vi "2013_01_03 Quality Motor.vi"(8 "Capture":bool, 9 "data":waveform(dbl)[](array[waveform]), 10 "File Path":path, 11 "Motor Typedef":T1={"Write"=FALSE, "Fail"=FALSE, "RPM"=0, "Motor"=enum."Maxon EC6 6V", "ESC"=enum."Phoenix", "Supply (V)"=0.0, "Test ID and Serial #"="", "Comments"="", "Elapsed Time"=0.0, "Counter"=0.0, "Torque (mNm)"=0.0, "Electrical Power (W)"=0.0, "Motor Efficiency"=0.0, "Mechanical Power (W)"=0.0, "Supply Power (W)"=0.0, "ESC Efficiency"=0.0, "No Load Speed"=0, "Stall Torque"=0.0, "Speed/Torque Gradient"=0, "Calcul"=FALSE, "Clear"=FALSE, "No Load Torque"=0.0} {"No Load Torque" format="%.3f"; "Stall Torque" format="%.3f"; "ESC Efficiency" format="%#_3g%%"; "Supply Power (W)" format="%.3f"; "Mechanical Power (W)" format="%.3f"; "Motor Efficiency" format="%#_3g%%"; "Electrical Power (W)" format="%.3f"; "Torque (mNm)" format="%.3f"; "Elapsed Time" format="%<%H:%M:%S>t"; "Supply (V)" format="%.2f"; "RPM" scale=0.0..60000.0}) -> (0 "Final Out":dynamicdata(graph), 3 "Motor Typedef Out":T1={"Write"=FALSE, "Fail"=FALSE, "RPM"=0, "Motor"=enum."Maxon EC6 6V", "ESC"=enum."Phoenix", "Supply (V)"=0.0, "Test ID and Serial #"="", "Comments"="", "Elapsed Time"=0.0, "Counter"=0.0, "Torque (mNm)"=0.0, "Electrical Power (W)"=0.0, "Motor Efficiency"=0.0, "Mechanical Power (W)"=0.0, "Supply Power (W)"=0.0, "ESC Efficiency"=0.0, "No Load Speed"=0, "Stall Torque"=0.0, "Speed/Torque Gradient"=0, "Calcul"=FALSE, "Clear"=FALSE, "No Load Torque"=0.0} {"No Load Torque" format="%.3f"; "Stall Torque" format="%.3f"; "ESC Efficiency" format="%#_3g%%"; "Supply Power (W)" format="%.3f"; "Mechanical Power (W)" format="%.3f"; "Motor Efficiency" format="%#_3g%%"; "Electrical Power (W)" format="%.3f"; "Torque (mNm)" format="%.3f"; "Elapsed Time" format="%<%H:%M:%S>t"; "Supply (V)" format="%.2f"; "RPM" scale=0.0..60000.0})   [LabVIEW 2013]
uses:
  Quality Type Def.ctl
  <vilib>/express/express shared/transition.llb/Dynamic To Waveform Array.vi
  <vilib>/express/express signal manip/GetorSetDDTAttributes/Set DDT Attributes/SetT0.vi
  <vilib>/express/express shared/transition.llb/Waveform Array To Dynamic.vi
  <vilib>/express/express signal manip/GetorSetDDTAttributes/Set DDT Attributes/Set DDT Properties.xnode
panel:
  in  "error in (no error)":errorcluster
  out "error out":errorcluster
  out "Saving Data":bool
  # "Fail"
  # "Fail"
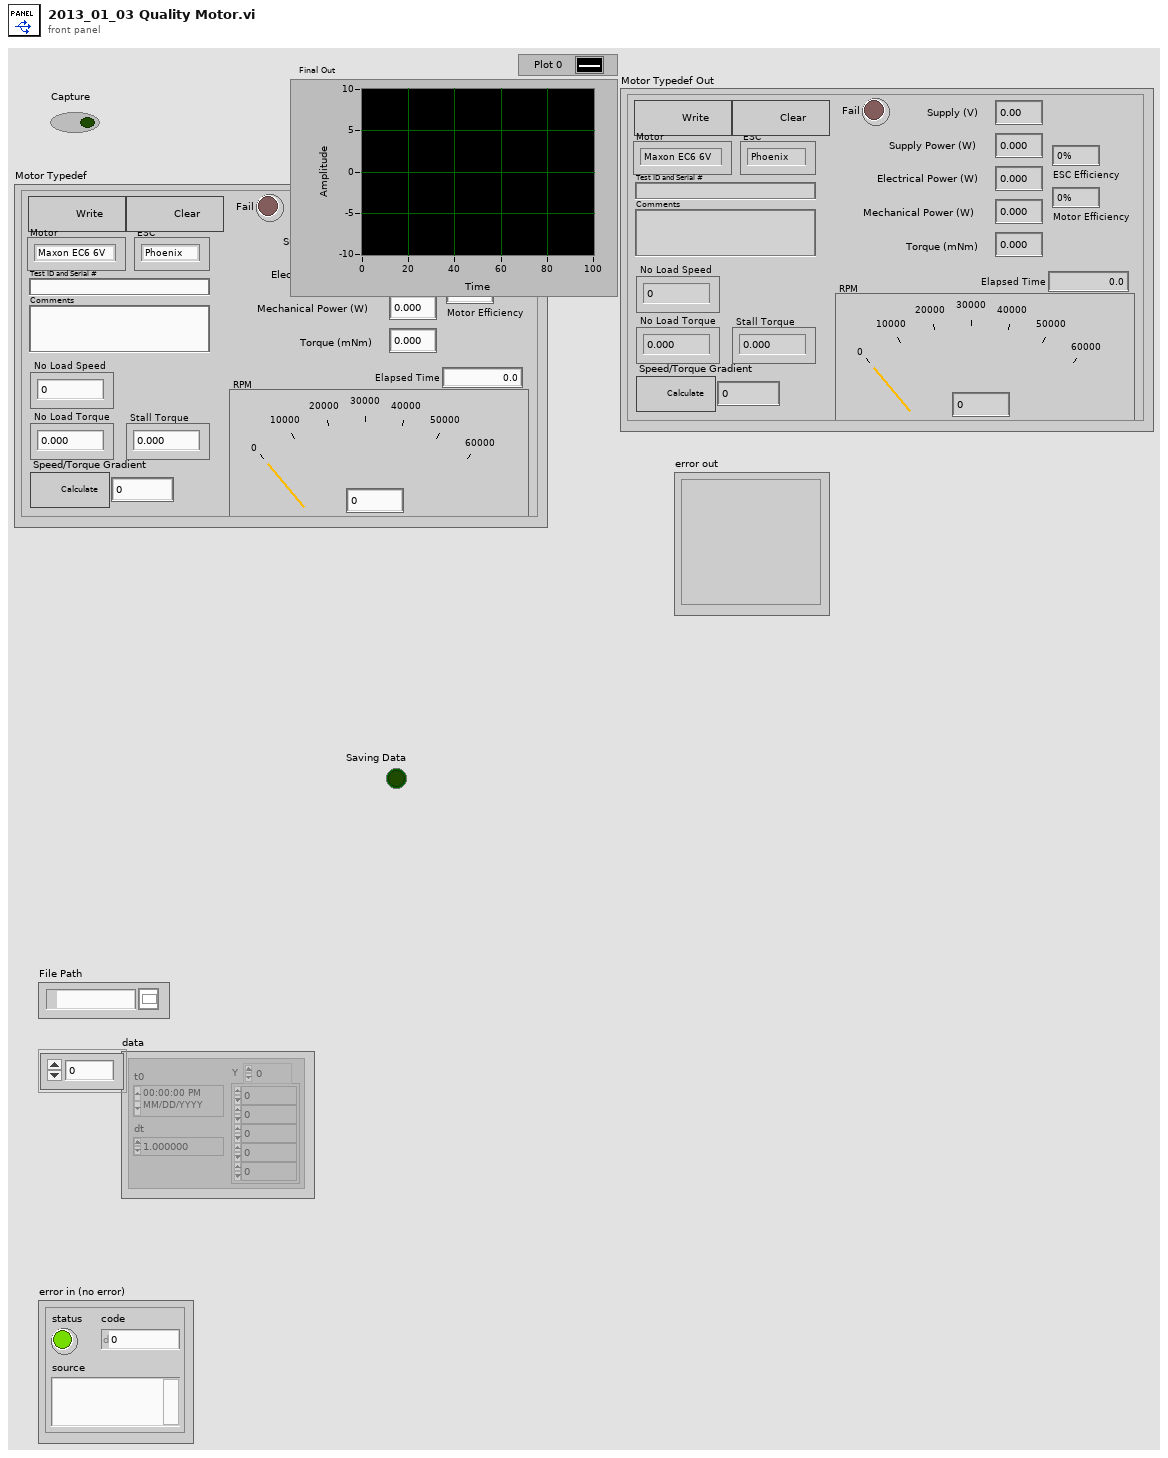
[diagram p1: front panel]
types:
  T1 = typedef "Quality Type Def.ctl" = cluster{"Write":bool, "Fail":bool, "RPM":u64, "Motor":enum16{"", "Maxon EC6 6V", "Maxon EC4 6V", "FH 0620 6V", "FH 0620 12V", "FH 0427 6V K2540"}, "ESC":enum16{"Phoenix", "Maxon", "FH 1801"}, "Supply (V)":dbl, "Test ID and Serial #":string, "Comments":string, "Elapsed Time":dbl, "Counter":dbl, "Torque (mNm)":dbl, "Electrical Power (W)":dbl, "Motor Efficiency":dbl, "Mechanical Power (W)":dbl, "Supply Power (W)":dbl, "ESC Efficiency":dbl, "No Load Speed":u32, "Stall Torque":dbl, "Speed/Torque Gradient":u32, "Calcul":bool, "Clear":bool, "No Load Torque":dbl}
  T2 = enum16{"", "Maxon EC6 6V", "Maxon EC4 6V", "FH 0620 6V", "FH 0620 12V", "FH 0427 6V K2540"}
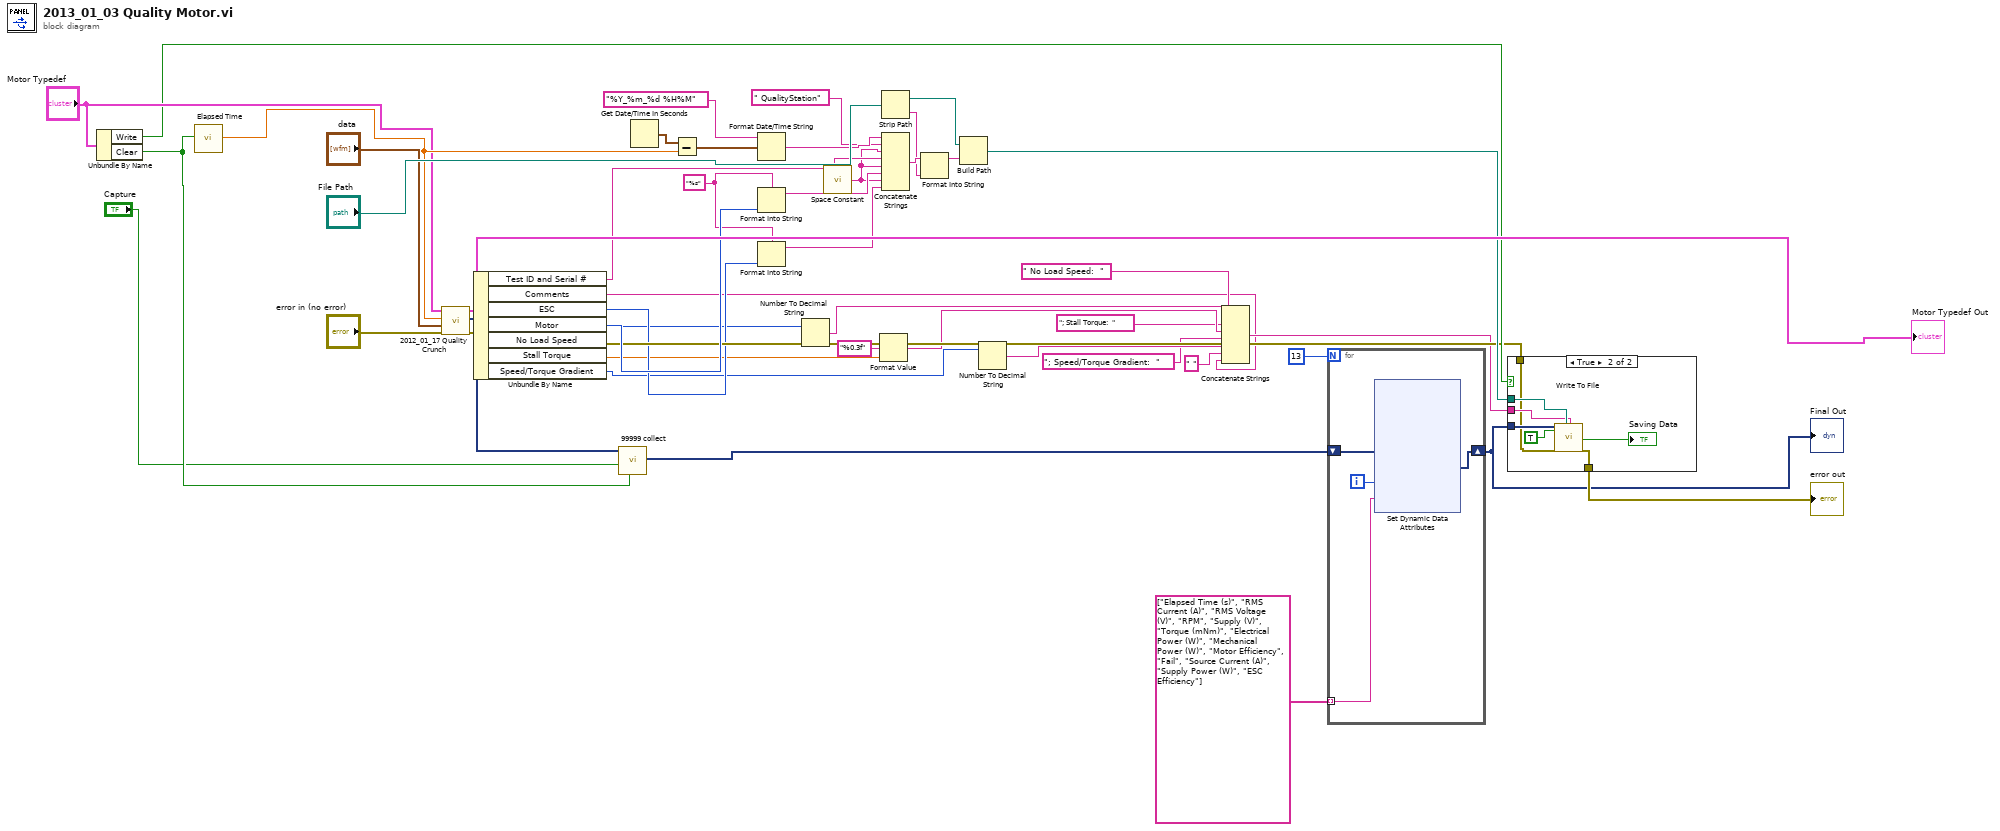
[diagram p0: block diagram]
diagram:
  w22 = "%s" ("format string")
  n1 = Unbundle By Name("Motor Typedef") -> ("Write"=w37:bool, "Clear"=w38:bool)
  n2 = call "Elapsed Time"("Reset"=w38) -> ("Elapsed Time (s)"=w41:dbl)  [unwired: 11 in, 7 out]
  n3 = call "2012_01_17 Quality Crunch.vi"("error in (no error)"="error in (no error)", "data"="data", "Elapsed Time (s)"=w41, "Motor In"="Motor Typedef") -> ("error out"=w19:errorcluster, "Dynamic Data Type"=w31:dynamicdata, "Motor Out"=w39:T1)  [unwired: 5 in]
  "Motor Typedef Out" <- w39
  n4 = Unbundle By Name(w39) -> ("Test ID and Serial #"=w21:string, "Comments"=w6:string, "ESC"=w17:enum16{"Phoenix", "Maxon", "FH 1801"}, "Motor"=w25:T2, "No Load Speed"=w16:u32, "Stall Torque"=w5:dbl, "Speed/Torque Gradient"=w15:u32)
  n5 = call "99999 collect"("Reset"=w38, "Enable"="Capture", "Signals"=w31) -> ("Collected Signals"=w18:dynamicdata)  [unwired: 7 in, 1 out]
  n6 = Get Date/Time In Seconds() -> (seconds since 1Jan1904=w28:timestamp)
  n7 = Subtract(x=w28, y=w41) -> (x-y=w27:timestamp)
  n8 = Format Date/Time String(time format string (%c)="%Y_%m_%d %H%M", seconds (now)=w27) -> (date/time string=w3:string)  [unwired: 1 in]
  n9 = Format Into String(format string=w22, w25) -> (resulting string=w24:string)  [unwired: 2 in, 1 out]
  n10 = Format Into String(format string=w22, w17) -> (resulting string=w23:string)  [unwired: 2 in, 1 out]
  n11 = Number To Decimal String(number=w16) -> (decimal integer string=w9:string)  [unwired: 1 in]
  n12 = call <vilib>:"Space Constant.vi"() -> ("String"=w20:string)
  n13 = Format Value(format string="%0.3f", value (0)=w5) -> (output string=w11:string)  [unwired: 1 in]
  n14 = Strip Path(path="File Path") -> (stripped path=w33:path, name=w34:string)
  n15 = Concatenate Strings(w3, " QualityStation" ("string"), w20, w21, w20, w24, w20, w23) -> (w35:string)
  n16 = Format Into String(initial string=w35, w34) -> (resulting string=w32:string)  [unwired: 2 in, 1 out]
  n17 = Build Path(base path=w33, name or relative path=w32) -> (appended path=w36:path)
  n18 = Number To Decimal String(number=w15) -> (decimal integer string=w13:string)  [unwired: 1 in]
  n19 = Concatenate Strings(" No Load Speed:  " ("string"), w9, "; Stall Torque:  " ("string"), w11, "; Speed/Torque Gradient:  " ("string"), w13, " " ("string"), w6) -> (w14:string)
  n20 = for {
    N: 13 -> [_]
    tunnel: string[] ["Elapsed Time (s)", "RMS Current (A)", "RMS Voltage (V)", "RPM", "Supply (V)", "Torque (mNm)", "Electrical Power (W)", "Mechanical Power (W)", "Motor Efficiency", "Fail", "Source Current (A)", "Supply Power (W)", "ESC Efficiency"] ("appended array") -> [w48] mode=indexing
    shift-right: [w49] -> w42
    shift-left: w18 -> [w47]
    i -> [w50]
    n21 = xnode "Set Dynamic Data Attributes"("Signals In"=w47, "Signal Index"=w50, "Signal Name"=w48) -> ("Signals Out"=w49:dynamicdata)  [unwired: 1 in, 1 out]
  }
  "Final Out" <- w42
  n22 = case shown="True" w37 {
    tunnel: w42 -> [_ w71]
    tunnel: w36 -> [_ w70]
    tunnel: w14 -> [_ w67]
    tunnel: [w64 w66] -> w45
    tunnel: w19 -> [w64 w65]
    frame False {
    }
    frame True {
      n23 = call "Write To File"("Signals"=w71, "Reset"=TRUE, "error in (no error)"=w65, "Filename"=w70, "Comment"=w67) -> ("Saving Data"=→"Saving Data":bool, "error out"=w66:errorcluster)  [unwired: 12 in, 1 out]
    }
  }
  "error out" <- w45
